vi "Version 1_Read Measurement Format.vi"(8 "error in":errorcluster, 9 "Totalizer Timer (Not connected internally)":enum32{"Disable", "Enable"}(radio)=enum."Enable", 11 "Address (A)":string="A") -> (0 "error out":errorcluster, 1 "Data - MAY NOT INCLUDE ALL OUTPUTS":T1, 2 "Missing data - Read Measurements.vi will not work!":bool, 3 "VISA Session Out":refnum<visa-resource-name>)   [LabVIEW 2016]
panel:
  in  "VISA Session In":refnum<visa-resource-name>="Alicat"
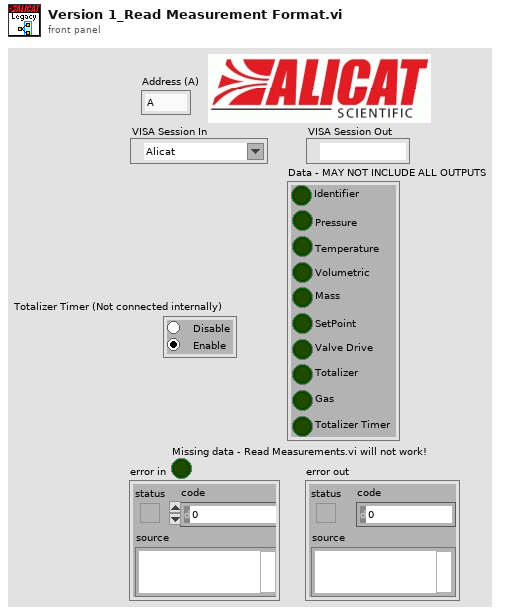
[diagram p1: front panel]
types:
  T1 = cluster{"Identifier":bool, "Pressure":bool, "Temperature":bool, "Volumetric":bool, "Mass":bool, "SetPoint":bool, "Valve Drive":bool, "Totalizer":bool, "Gas":bool, "Totalizer Timer":bool}
  T2 = typedef "Data Frame.ctl" = cluster{"Absolute Pressure":bool, "Gauge/Diff. Pressure":bool, "Barometric Pressure":bool, "Temperature":bool, "Volumetric":bool, "Mass":bool, "Setpoint":bool, "Valve Drive":bool, "Totalizer":bool, "Totalizer Timer":bool, "Totalizer Average Flow":bool, "Totalizer Peak Flow":bool, "Gas Selected":bool, "Tot. Timer Format":u16}
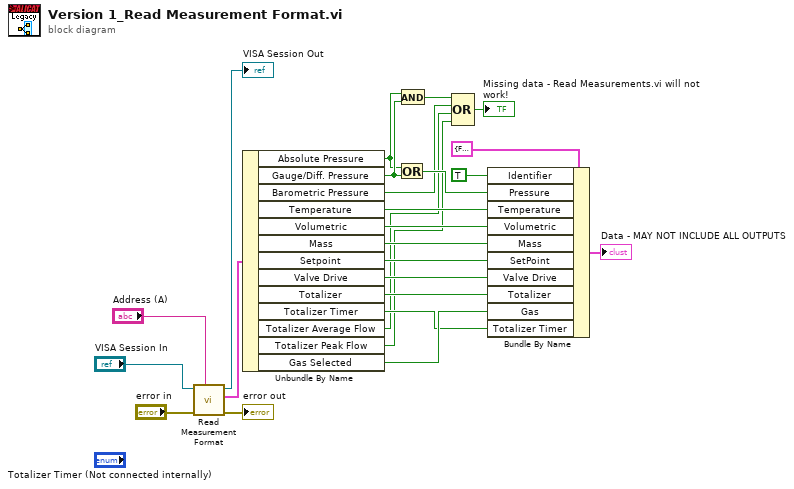
[diagram p0: block diagram]
diagram:
  n1 = call "Read Measurement Format.vi"("Unit ID (A)"="Address (A)", "error in"="error in", "VISA Session In"="VISA Session In") -> ("error out"=→"error out":errorcluster, "Data Frame Format"=w17:T2, "VISA Session Out"=→"VISA Session Out":refnum<visa-resource-name>)  [unwired: 6 in]
  n2 = Unbundle By Name(w17) -> ("Absolute Pressure"=w3:bool, "Gauge/Diff. Pressure"=w4:bool, "Barometric Pressure"=w5:bool, "Temperature"=w15:bool, "Volumetric"=w14:bool, "Mass"=w13:bool, "Setpoint"=w12:bool, "Valve Drive"=w11:bool, "Totalizer"=w10:bool, "Totalizer Timer"=w8:bool, "Totalizer Average Flow"=w6:bool, "Totalizer Peak Flow"=w7:bool, "Gas Selected"=w9:bool)
  n3 = Or(x=w3, y=w4) -> (x .or. y?=w16:bool)
  n4 = And(x=w3, y=w4) -> (x .and. y?=w2:bool)
  n5 = Compound Arithmetic op=OR(w2, w5, w6, w7) -> (→"Missing data - Read Measurements.vi will not work!":bool)
  n6 = Bundle By Name(cluster=T1 {"Identifier"=FALSE, "Pressure"=FALSE, "Temperature"=FALSE, "Volumetric"=FALSE, "Mass"=FALSE, "SetPoint"=FALSE, "Valve Drive"=FALSE, "Totalizer"=FALSE, "Gas"=FALSE, "Totalizer Timer"=FALSE} ("Data"), "Identifier"=TRUE, "Pressure"=w16, "Temperature"=w15, "Volumetric"=w14, "Mass"=w13, "SetPoint"=w12, "Valve Drive"=w11, "Totalizer"=w10, "Gas"=w9, "Totalizer Timer"=w8) -> (→"Data - MAY NOT INCLUDE ALL OUTPUTS":T1)
